vi "Close.vi"(8 "error in (no error)":errorcluster, 11 "Device in":refnum<class "Device.lvclass">) -> (0 "error out":errorcluster, 3 "Device out":refnum<class "Device.lvclass">)   [LabVIEW 2019, in "Device.lvclass"]
uses:
  Device.lvclass
  Device.lvclass/Device.ctl
  SV_Puplisher_class/SV_Publisher.lvclass
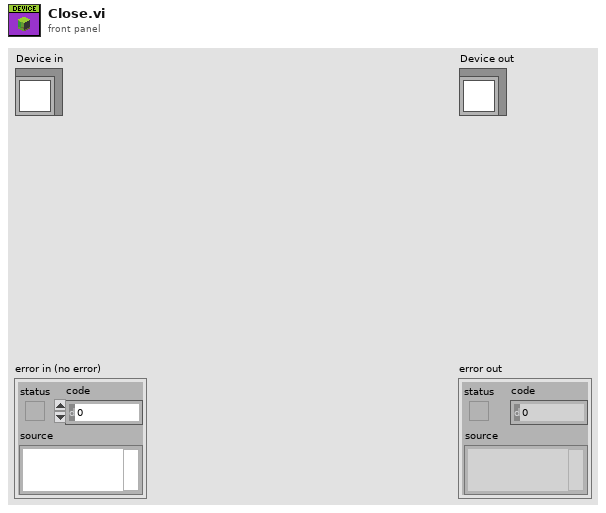
[diagram p1: front panel]
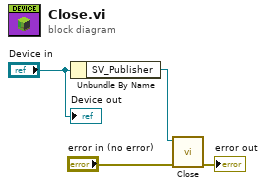
[diagram p0: block diagram]
diagram:
  n1 = Unbundle By Name("Device in") -> ("SV_Publisher"=w3:refnum<class "SV_Publisher.lvclass">)
  n2 = call "Close.vi"("error in (no error)"="error in (no error)", "SV_Publisher in"=w3) -> ("error out"=→"error out":errorcluster)  [unwired: 8 in, 1 out]
  "Device out" <- "Device in"
